vi "8bit sync-Gen patches montage C.vi"(0 "8-bit Image refs cluster":T1, 1 "max value":dbl, 3 "Channel":enum16{"Green", "Red"}(ring)=enum."Red", 4 "Global cycle number among all trials":i32, 5 "error in (no error)":errorcluster) -> (16 "U8 Image (Montage)":T2, 19 "error out":errorcluster)   [LabVIEW 2020]
uses:
  <vilib>/vision/Image Controls.llb/IMAQ Image.ctl
  Typedefs/8bit sync-IMAQ image refs.ctl
  Typedefs/Read Write Enum.ctl
  Globals/gl_8-bit montage window ctrl refs.vi
  <vilib>/vision/NI_Vision_Development_Module.lvlib
panel:
  out "max value 3":u8
  out "max value 2":dbl
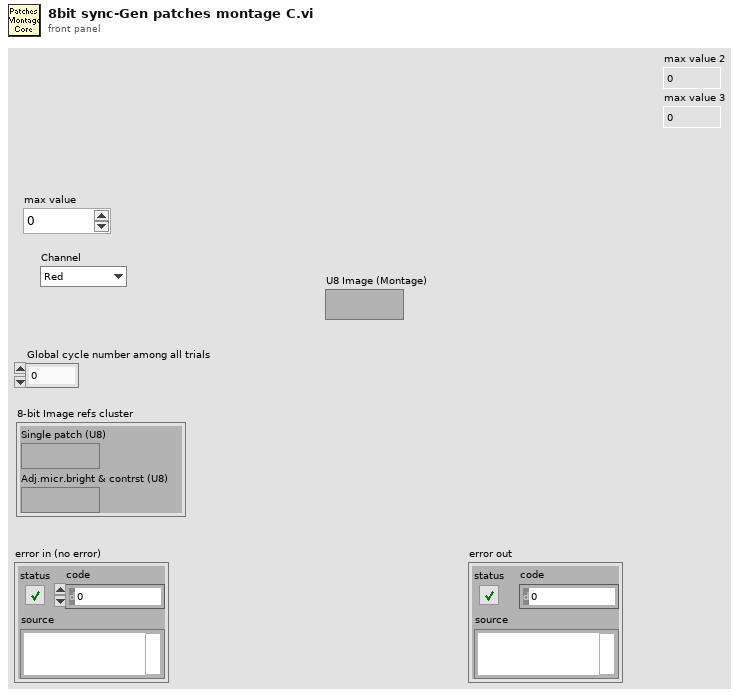
[diagram p1: front panel]
types:
  T1 = typedef "8bit sync-IMAQ image refs.ctl" = cluster{"Single patch (U8)":T2, "Adj.micr.bright & contrst (U8)":T2}
  T2 = typedef "IMAQ Image.ctl" = refnum<image>
  T3 = typedef "Read Write Enum.ctl" = enum16{"Read", "Write"}
  T4 = typedef "8-bit video export window ctrl refs.ctl" = cluster{"This VI":refnum<vi>, "Add speed data":refnum<vi>, "Add camera videos":refnum<vi>, "Stop button":refnum<vi>, "Camera Video Adjustments":refnum<vi>, "Microscope Image Adjustments":refnum<vi>, "Execute":refnum<vi>, "Codec":refnum<vi>, "Channel to load":refnum<vi>, "Speed graph behaviour":refnum<vi>, "Include speed graph":refnum<vi>, "Number of rows to generate":refnum<vi>, "Path":refnum<vi>}
  T5 = typedef "Patch viewer internal cluster.ctl" = cluster{"Image ref":T2, "Variable Length ?":bool, "Coordinates of montage positions":cluster{"X\n\nY":i32[]}[], "TDMS refs":refnum<k34>[], "Frames info":cluster{"Frame numbers used":i32[], "Frame position index":i32[]}, "Number of trials":i32, "Cycles in single trial":i32, "Total number of cycles":i32, "Number of patches":i32, "Pixels in a cycle":i32, "Patches info array":cluster{"Pixels in a patch":i32, "X size of patch":i32, "Y size of patch":i32}[], "Start Coordinates":cluster{"X start":i32, "Y start":i32, "Z start":i32}[], "Stop Coordinates":cluster{"X stop":i32, "Y stop":i32, "Z stop":i32}[], "VL Image Refs":T2[], "error":errorcluster}
  T6 = cluster{"Frame numbers used":i32[], "Frame position index":i32[]}
  T7 = cluster{"Pixels in a patch":i32, "X size of patch":i32, "Y size of patch":i32}[]
  T8 = typedef "Bright-Contr-Gamma cluster.ctl" = cluster{"Brightness":sgl, "Contrast":sgl, "Gamma":sgl}
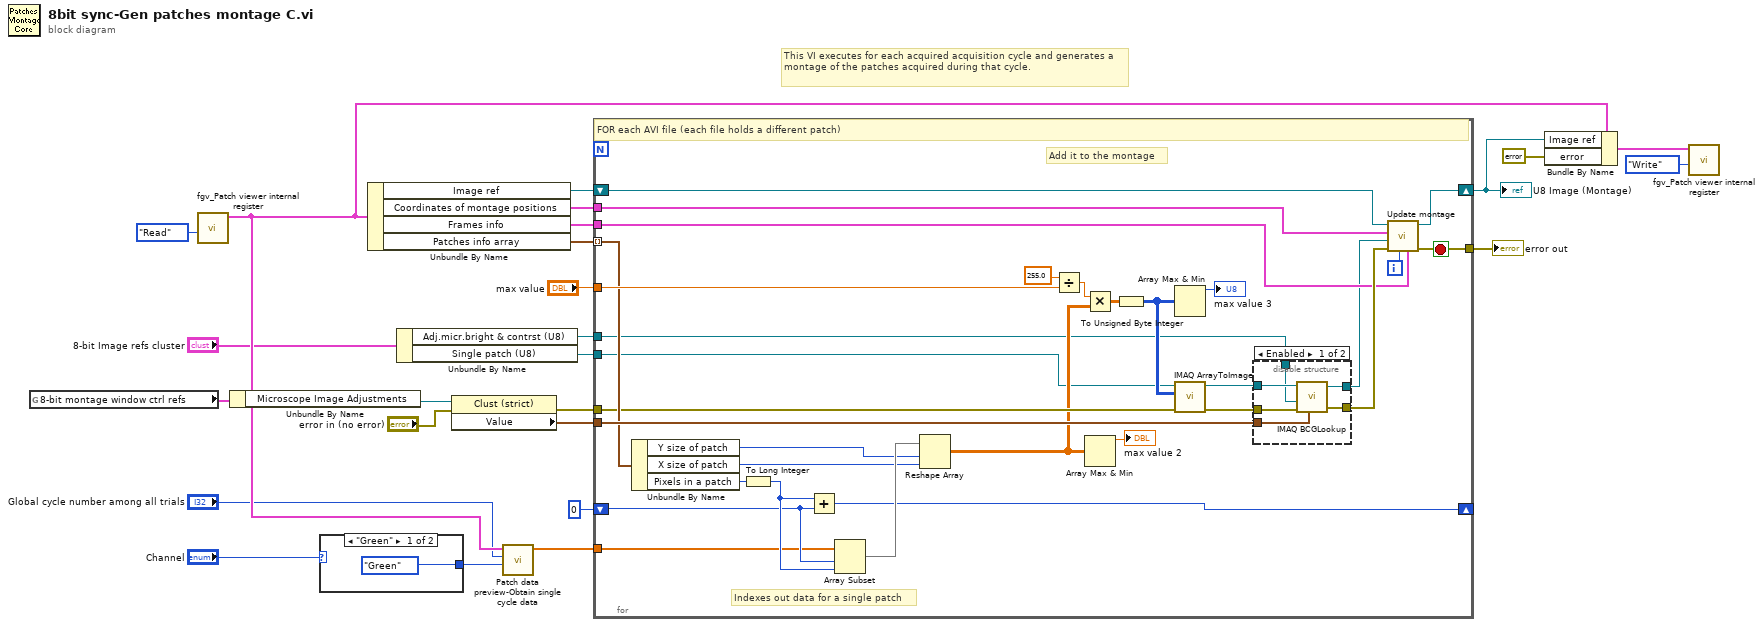
[diagram p0: block diagram]
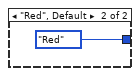
[diagram p2: hidden frame]
diagram:
  # "This VI executes for each acquired acquisition cycle and generates a montage of the patches acquired during that cycle."
  n1 = global read "gl_8-bit montage window ctrl refs.vi" "8-bit montage window ctrl refs"() -> (w23:T4)
  n2 = call "fgv_Patch viewer internal register.vi"("Function"=Read_Write_Enum."Read") -> ("Registered setup"=w5:T5)  [unwired: 10 in]
  n3 = Unbundle By Name(w23) -> ("Microscope Image Adjustments"=w24:refnum<vi>)
  n4 = case shown="\"Green\"" "Channel" {
    tunnel: [enum16{"Red", "Green"}."Green" ("Channel to load") enum16{"Red", "Green"}."Red" ("Channel to load")] -> w6
    frame "Green" {
    }
    frame "Red", Default {
    }
  }
  n5 = Unbundle By Name(w5) -> ("Image ref"=w16:T2, "Coordinates of montage positions"=w17:cluster{"X\n\nY":i32[]}[], "Frames info"=w15:T6, "Patches info array"=w14:T7)
  n6 = Unbundle By Name("8-bit Image refs cluster") -> ("Adj.micr.bright & contrst (U8)"=w1:T2, "Single patch (U8)"=w2:T2)
  n7 = property class="Clust (strict)"(reference=w24, error in="error in (no error)") -> (error out=w20:errorcluster, "Value"=w21:T8)  [unwired: 1 out]
  n8 = call "Patch data preview-Obtain single cycle data.vi"("Channel to load"=w6, "Global cycle number among all trials"="Global cycle number among all trials", "Register cluster"=w5) -> ("Data from single channel single cycle"=w8:dbl[])  [unwired: 6 in, 2 out]
  n9 = for {
    tunnel: [w54] -> w25
    tunnel: w20 -> [w32]
    shift-right: [w55] -> w11
    shift-left: w16 -> [w58]
    tunnel: w17 -> [w57]
    tunnel: w21 -> [w52]
    tunnel: w1 -> [w29]
    tunnel: "max value" -> [w47]
    tunnel: w2 -> [w28]
    tunnel: w15 -> [w42]
    tunnel: w14 -> [w36] mode=indexing
    shift-right: [w34] -> _
    shift-left: 0 -> [w35]
    tunnel: w8 -> [w33]
    i -> [w56]
    stop <- w54 stop-if-true
    # "Indexes out data for a single patch"
    # "Add it to the montage"
    # "FOR each AVI file (each file holds a different patch)"
    n10 = Unbundle By Name(w36) -> ("Y size of patch"=w38:i32, "X size of patch"=w37:i32, "Pixels in a patch"=w41:i32)
    n11 = To Long Integer(number=w41) -> (32bit integer=w40:i32)
    n12 = Add(x=w40, y=w35) -> (x+y=w34:i32)
    n13 = Array Subset "Array Subset"(array=w33, index=w35, length=w40) -> (w39:dbl[])
    n14 = Reshape Array(w39, w38, w37) -> (w31:dbl[][])
    n15 = Divide(x=255.0 ("Numeric"), y=w47) -> (x/y=w49:dbl)
    n16 = Multiply(x=w49, y=w31) -> (x*y=w50:dbl[][])
    n17 = Array Max & Min(array=w31) -> (max value=→"max value 2":dbl)  [unwired: 3 out]
    n18 = To Unsigned Byte Integer(number=w50) -> (unsigned 8bit integer=w45:u8[][])
    n19 = Array Max & Min(array=w45) -> (max value=→"max value 3":u8)  [unwired: 3 out]
    n20 = call "IMAQ ArrayToImage"("error in (no error)"=w32, "Image Pixels (U8)"=w45, "Image"=w28) -> ("error out"=w46:errorcluster, "Image Out"=w51:T2)  [unwired: 7 in]
    n21 = disable-structure shown="Enabled" {
      disable-tunnel: [w64 w66] -> w30
      disable-tunnel: [w63 w65] -> w53
      disable-tunnel: w46 -> [w62 w65]
      disable-tunnel: w52 -> [w59 _]
      disable-tunnel: w51 -> [w61 w66]
      disable-tunnel: w29 -> [w60 _]
      frame Enabled {
        n22 = call "IMAQ BCGLookup"("Image Src"=w61, "BCG Values"=w59, "Image Dst"=w60, "error in (no error)"=w62) -> ("Image Dst Out"=w64:T2, "error out"=w63:errorcluster)  [unwired: 3 in]
      }
      frame Disabled {
      }
    }
    n23 = call "Update montage.vi"("Frames info"=w42, "Frame's rel. index"=w56, "Error in"=w53, "Single patch image"=w30, "Coordinates of montage positions"=w57, "Image (Montage)"=w58) -> ("error out"=w54:errorcluster, "Image (Montage)"=w55:T2)  [unwired: 4 in]
  }
  "error out" <- w25
  "U8 Image (Montage)" <- w11
  n24 = Bundle By Name(cluster=w5, "Image ref"=w11, "error"=errorcluster {"status"=FALSE, "code"=0, "source"=""}) -> (w10:T5)
  n25 = call "fgv_Patch viewer internal register.vi"("Function"=Read_Write_Enum."Write", "Registered setup"=w10) -> ()  [unwired: 9 in, 1 out]
